vi "2.A.3-Spoof Relative Wind.vi"(3 "Wind Speed":dbl, 4 "Wind Angle":dbl, 5 "Velocity (3 array)":dbl[](array[numeric])) -> (0 "Perceived Wind":cluster{"X Position":dbl, "Y Position":dbl}, 1 "Global Wind":cluster{"X Position":dbl, "Y Position":dbl}, 2 "Orientation":cluster{"X Position":dbl, "Y Position":dbl})   [LabVIEW 2011]
uses:
  <vilib>/Analysis/_algsub.llb/Real Vector Norm.vi
  <vilib>/Analysis/baseanly.llb/Real Dot Product.vi
  <vilib>/Analysis/NI_AALPro.lvlib
  <vilib>/Analysis/NI_AALBase.lvlib
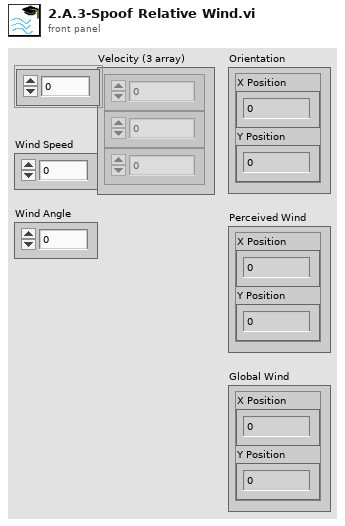
[diagram p1: front panel]
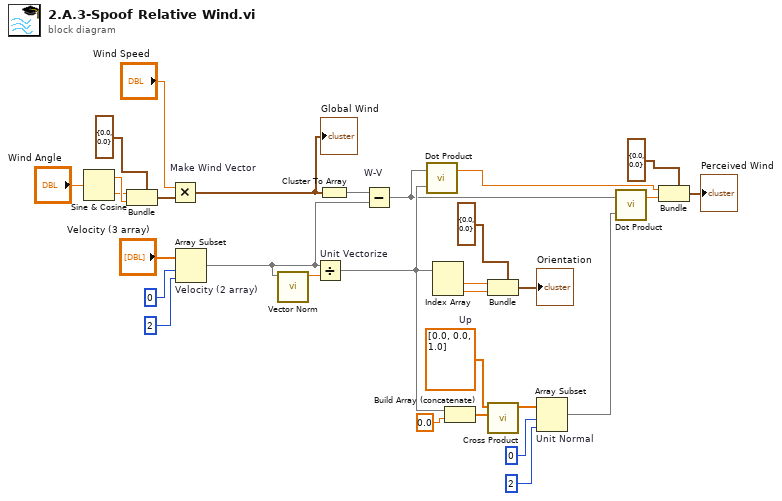
[diagram p0: block diagram]
diagram:
  w1 = dbl[] [0.0, 0.0, 1.0]  # Up
  n1 = Sine & Cosine(0:"Wind Angle") -> (1:w16:dbl, 2:w15:dbl)
  n2 = Bundle(cluster=cluster{"X Position":dbl, "Y Position":dbl} {"X Position"=0.0, "Y Position"=0.0} ("Robot Location"), "X Position"=w15, "Y Position"=w16) -> (w17:cluster{"X Position":dbl, "Y Position":dbl})
  n3 = Multiply "Make Wind Vector"(x="Wind Speed", y=w17) -> (x*y=w21:cluster{"X Position":dbl, "Y Position":dbl})
  "Global Wind" <- w21
  n4 = Array Subset "Velocity (2 array)"(array="Velocity (3 array)", index=0, length=2) -> (w11:dbl[])
  n5 = call-poly <vilib>:"Vector Norm.vi"("Input Vector"=w11) -> ("norm"=w30:dbl)  [unwired: 9 in, 1 out]
  n6 = Divide "Unit Vectorize"(x=w11, y=w30) -> (x/y=w10:dbl[])
  n7 = Cluster To Array(cluster=w21) -> (array=w26:dbl[])
  n8 = Subtract "W-V"(x=w26, y=w11) -> (x-y=w5:dbl[])
  n9 = call-poly <vilib>:"Dot Product.vi"("Y Vector"=w10, "X Vector"=w5) -> ("X * Y"=w28:dbl)  [unwired: 1 out]
  n10 = Index Array(array=w10) -> (element #1=w23:dbl, element #2=w24:dbl)  [unwired: 2 in]
  n11 = Build Array (concatenate)(w10, 0.0) -> (w2:dbl[])
  n12 = Bundle(cluster=cluster{"X Position":dbl, "Y Position":dbl} {"X Position"=0.0, "Y Position"=0.0} ("Robot Location"), "X Position"=w23, "Y Position"=w24) -> (→"Orientation":cluster{"X Position":dbl, "Y Position":dbl})
  n13 = call <vilib>:"Cross Product.vi"("B Vector"=w2, "A Vector"=w1) -> ("Cross Product"=w6:dbl[])  [unwired: 8 in, 1 out]
  n14 = Array Subset "Unit Normal"(array=w6, index=0, length=2) -> (w4:dbl[])
  n15 = call-poly <vilib>:"Dot Product.vi"("Y Vector"=w4, "X Vector"=w5) -> ("X * Y"=w3:dbl)  [unwired: 1 out]
  n16 = Bundle(cluster=cluster{"X Position":dbl, "Y Position":dbl} {"X Position"=0.0, "Y Position"=0.0} ("Perceived Wind"), "X Position"=w28, "Y Position"=w3) -> (→"Perceived Wind":cluster{"X Position":dbl, "Y Position":dbl})
